vi "PH_SystemInformation.get Enabling State.vi"(0 "i ref in":refnum<vi>, 2 "Wanted State":T1(ring), 5 "error in (no error)":errorcluster) -> (14 "i ref out":refnum<vi>, 17 "Enabling State":T2 items=["no info", "not disabled", "disabled"], 19 "error out":errorcluster)   [LabVIEW 2014, in "PH_SystemInformation.lvlib"]
doc: "By this VI one gets the requested enabling state."
uses:
  PH_SystemInformation.lvlib
  PH_SystemInformationEnabling State.ctl
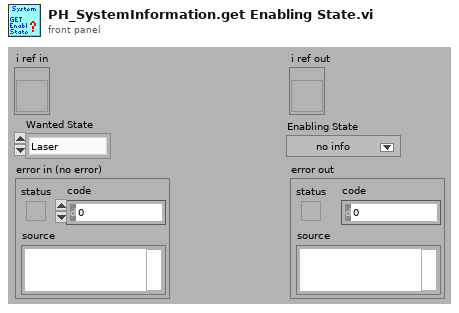
[diagram p1: front panel]
types:
  T1 = enum16{"Laser", "PreAmp", "MainAmp", "Exp 1", "Exp 2", "Exp 3", "Exp 4"}
  T2 = typedef "PH_SystemInformation.lvlib/PH_SystemInformationEnabling State.ctl" = i32
  T3 = typedef "PH_SystemInformation.lvlib/PH_SystemInformation.i attribute.ctl" = cluster{"Laser Enabling":cluster{"GUI Ref":refnum<vi>, "Enabling State":T2}, "PreAmp Enabling":cluster{"GUI Ref":refnum<vi>, "Enabling State":T2}, "MainAmp Enabling":cluster{"GUI Ref":refnum<vi>, "Enabling State":T2}, "Emergency Off":cluster{"GUI Ref":refnum<vi>, "State":enum16{"no info", "off/false", "Alarm"}}, "Enabling Exp. 1":cluster{"GUI Ref":refnum<vi>, "Enabling State":T2}, "Enabling Exp. 2":cluster{"GUI Ref":refnum<vi>, "Enabling State":T2}, "Enabling Exp. 3":cluster{"GUI Ref":refnum<vi>, "Enabling State":T2}, "Enabling Exp. 4":cluster{"GUI Ref":refnum<vi>, "Enabling State":T2}, "Timing Mode":cluster{"GUI Ref":refnum<vi>, "PHELIX_Timing_Mode":enum32{"10 Hz", "0.5 Hz", "Shot"}}}
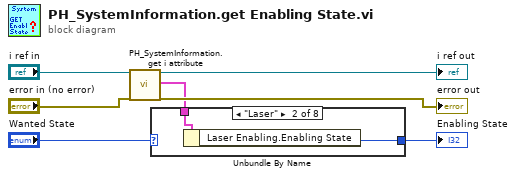
[diagram p0: block diagram]
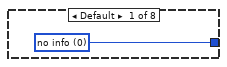
[diagram p2: hidden frame]
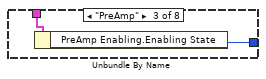
[diagram p3: hidden frame]
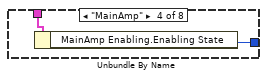
[diagram p4: hidden frame]
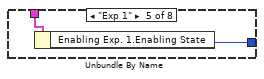
[diagram p5: hidden frame]
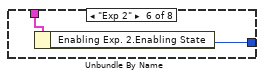
[diagram p6: hidden frame]
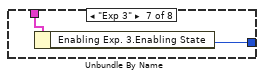
[diagram p7: hidden frame]
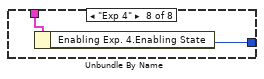
[diagram p8: hidden frame]
diagram:
  n1 = call "PH_SystemInformation.get i attribute.vi"("i ref in"="i ref in", "error in (no error)"="error in (no error)") -> ("i ref out"=→"i ref out":refnum<vi>, "i attribute"=w3:T3, "error out"=→"error out":errorcluster)  [unwired: 15 in]
  n2 = case shown="\"Laser\"" "Wanted State" {
    tunnel: w3 -> [_ w10 w12 w14 w16 w18 w20 w22]
    tunnel: [w8 w9 w11 w13 w15 w17 w19 w21] -> w2
    frame Default {
      w8 = T2 0 items=["no info", "not disabled", "disabled"] ("Enabling State")
    }
    frame "Laser" {
      n3 = Unbundle By Name(w10) -> ("Laser Enabling.Enabling State"=w9:T2)
    }
    frame "PreAmp" {
      n4 = Unbundle By Name(w12) -> ("PreAmp Enabling.Enabling State"=w11:T2)
    }
    frame "MainAmp" {
      n5 = Unbundle By Name(w14) -> ("MainAmp Enabling.Enabling State"=w13:T2)
    }
    frame "Exp 1" {
      n6 = Unbundle By Name(w16) -> ("Enabling Exp. 1.Enabling State"=w15:T2)
    }
    frame "Exp 2" {
      n7 = Unbundle By Name(w18) -> ("Enabling Exp. 2.Enabling State"=w17:T2)
    }
    frame "Exp 3" {
      n8 = Unbundle By Name(w20) -> ("Enabling Exp. 3.Enabling State"=w19:T2)
    }
    frame "Exp 4" {
      n9 = Unbundle By Name(w22) -> ("Enabling Exp. 4.Enabling State"=w21:T2)
    }
  }
  "Enabling State" <- w2
